vi "Process-received-message.vi"(8 "error in (no error)":errorcluster, 10 "Message":refnum<class "Message.lvclass">, 11 "Client in":T1) -> (0 "error out":errorcluster, 3 "Client out":T1)   [LabVIEW 2013, in "Module-communication.lvlib" / "Client.lvclass"]
uses:
  Client.lvclass
  Object-reference.ctl
  Messages/Message.lvclass
  Allowed-modules.ctl
  Messages/Message.lvclass/Message.ctl
  Messages/Read Message type.vi
  Messages/Read Sender type.vi
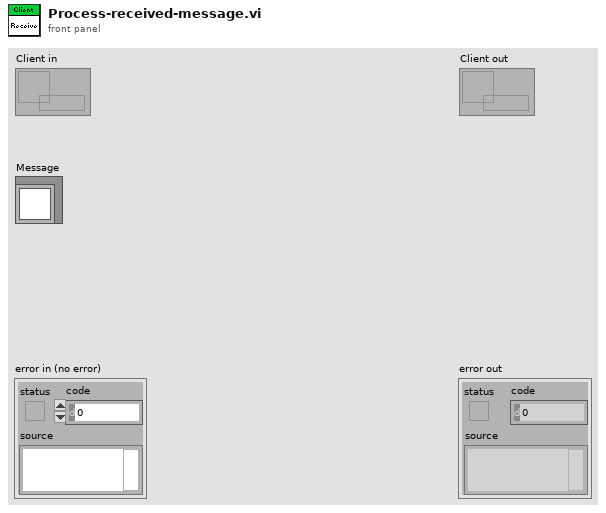
[diagram p1: front panel]
types:
  T1 = typedef "Module-communication.lvlib/Client.lvclass/Object-reference.ctl" = refnum<data-value>
  T2 = typedef "Module-communication.lvlib/Client.lvclass/Allowed-modules.ctl" = enum16{"Server", "All", "BeamControl", "PowderDeposition", "StrategyParser", "CameraVision", "MaterialCharacterization", "StatusMonitor", "SLMSimulation", "LaserCharacterization"}
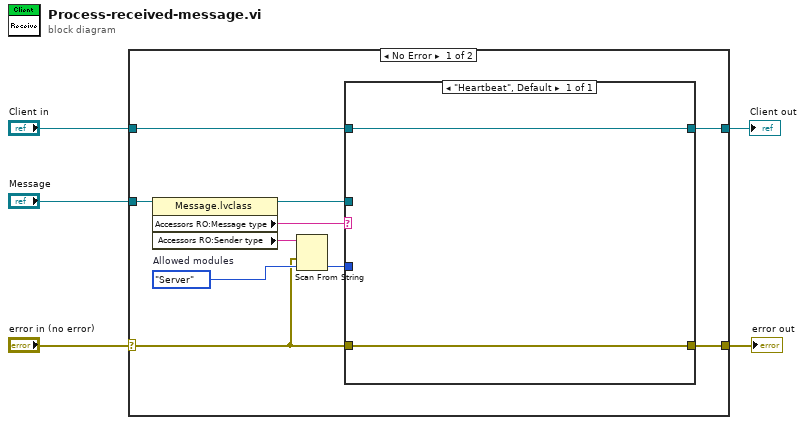
[diagram p0: block diagram]
diagram:
  n1 = case shown="No Error" "error in (no error)" {
    selector: "error in (no error)" -> [w13 w19]
    tunnel: [w12 w19] -> w4
    tunnel: [w7 w18] -> w2
    tunnel: "Client in" -> [w11 w18]
    tunnel: "Message" -> [w15 _]
    frame No Error {
      w14 = Allowed-modules."Server"  # Allowed modules
      n2 = property class="Message.lvclass"(reference=w15) -> (reference out=w6:refnum<class "Message.lvclass">, "Accessors RO:Message type"=w9:string, "Accessors RO:Sender type"=w10:string)  [unwired: 1 in, 1 out]
      n3 = Scan From String(input string=w10, error in=w13, default 1=w14) -> (output 1=w8:T2)  [unwired: 2 in, 3 out]
      n4 = case shown="\"Heartbeat\", Default" w9 {
        tunnel: w13 -> [w17]
        tunnel: [w17] -> w12
        tunnel: w11 -> [w16]
        tunnel: w8 -> [_]
        tunnel: [w16] -> w7
        tunnel: w6 -> [_]
        frame "Heartbeat", Default {
        }
      }
    }
    frame Error {
    }
  }
  "error out" <- w4
  "Client out" <- w2
